vi "Get Size of Data from TD - Variant With Attributes - Returns Correct Size.vi"() -> ()   [LabVIEW 2017, in "Composition.Tests.lvlib"]
uses:
  Composition.Tests.lvlib
  <vilib>/addons/_JKI Toolkits/Caraya/classes/Assert/Assert Equal Value_Variant.vi
  Composition/Composition.lvlib
  <vilib>/addons/_JKI Toolkits/Caraya/classes/Test/Test.lvclass
  <vilib>/addons/_JKI Toolkits/Caraya/classes/Assert/Assert.lvclass
panel:
  out "error out":errorcluster
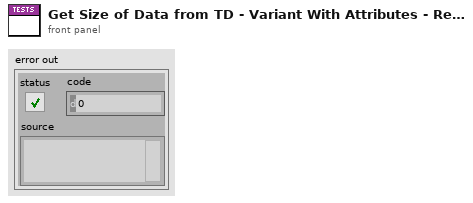
[diagram p1: front panel]
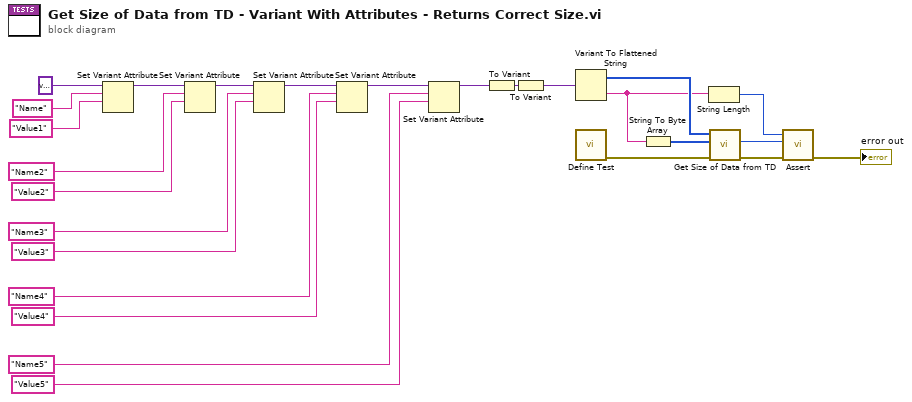
[diagram p0: block diagram]
diagram:
  n1 = Set Variant Attribute(Variant=variant, name="Name", value="Value1") -> (Variant out=w14:variant)  [unwired: 1 in, 2 out]
  n2 = Set Variant Attribute(Variant=w14, name="Name2", value="Value2") -> (Variant out=w10:variant)  [unwired: 1 in, 2 out]
  n3 = Set Variant Attribute(Variant=w10, name="Name3", value="Value3") -> (Variant out=w9:variant)  [unwired: 1 in, 2 out]
  n4 = Set Variant Attribute(Variant=w9, name="Name4", value="Value4") -> (Variant out=w4:variant)  [unwired: 1 in, 2 out]
  n5 = Set Variant Attribute(Variant=w4, name="Name5", value="Value5") -> (Variant out=w3:variant)  [unwired: 1 in, 2 out]
  n6 = To Variant(anything=w3) -> (Variant=w13:variant)
  n7 = To Variant(anything=w13) -> (Variant=w25:variant)
  n8 = Variant To Flattened String(Variant=w25) -> (data string=w18:string, 1:w19:i16[])
  n9 = call <vilib>:"Define Test.vi"() -> ("error out"=w24:errorcluster)  [unwired: 10 in, 1 out]
  n10 = String To Byte Array(string=w18) -> (unsigned byte array=w26:u8[])
  n11 = String Length(string=w18) -> (length=w20:i32)
  n12 = call "Get Size of Data from TD.vi"("error in (no error)"=w24, "Data String"=w26, "Type Descriptor"=w19) -> ("error out"=w23:errorcluster, "Size of Data"=w22:i32)  [unwired: 7 in]
  n13 = call-poly <vilib>:"Assert.vi"("error in (no error)"=w23, "Y"=w22, "X"=w20) -> ("error out"=→"error out":errorcluster)  [unwired: 7 in, 1 out]
